vi "get Application Ini File.vi"() -> (3 "Application Ini File":path)   [LabVIEW 2015]
uses:
  Re-use Libraries/Utility/Utility.lvlib
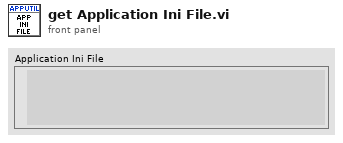
[diagram p1: front panel]
types:
  T1 = typedef "Utility.lvlib/App Paths.ctl" = cluster{"App Ini File":path, "App Data Dir":path, "Config Dir":path, "App Root Dir":path}
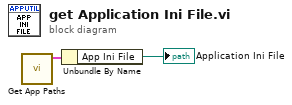
[diagram p0: block diagram]
diagram:
  n1 = call "Get App Paths.vi"() -> ("Paths"=w2:T1)  [unwired: 10 in, 1 out]
  n2 = Unbundle By Name(w2) -> ("App Ini File"=→"Application Ini File":path)
